vi "Database Recordset Upadate.vi"(8 "error in (no error)":errorcluster caption="错误输入（无错误）", 9 "Values":variant, 10 "Fields":variant, 11 "Database Recordset 输入":refnum<class "Database Recordset.lvclass"> caption="DNL_LabVIEW Object in") -> (0 "error out":errorcluster caption="错误输出", 3 "Database Recordset 输出":refnum<class "Database Recordset.lvclass"> caption="DNL_LabVIEW Object out")   [LabVIEW 2011, in "Database Recordset.lvclass"]
uses:
  Database Recordset.lvclass
  Database Recordset.lvclass/Database Recordset.ctl
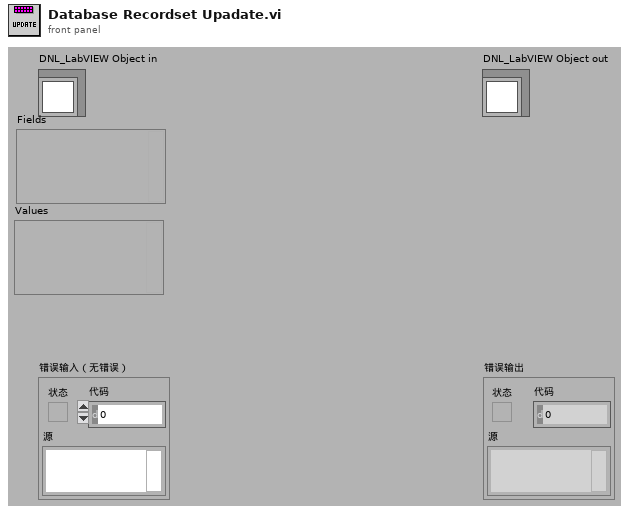
[diagram p1: front panel]
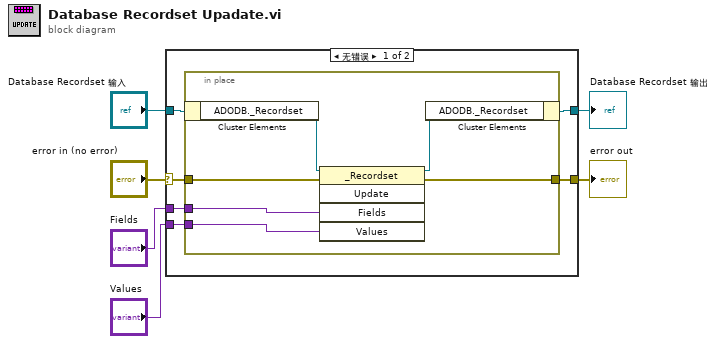
[diagram p0: block diagram]
diagram:
  n1 = case shown="无错误" "error in (no error)" {
    selector: "error in (no error)" -> [w8 w20]
    tunnel: [w7 w20] -> w5
    tunnel: [w9 w19] -> w3
    tunnel: "Database Recordset 输入" -> [w12 w19]
    tunnel: "Fields" -> [w11 _]
    tunnel: "Values" -> [w10 _]
    frame No Error {
      n2 = in-place {
        in-place-border: w11 -> [w16]
        in-place-border: w10 -> [w15]
        in-place-border: w8 -> [w14]
        in-place-border: [w13] -> w7
        n3 = in-place-cluster #1(w12) -> ("ADODB._Recordset"=w18:refnum<k7>)
        n4 = invoke class="_Recordset" method="Update"(reference=w18, error in=w14, "Fields"=w16, "Values"=w15) -> (reference out=w17:refnum<k7>, error out=w13:errorcluster)  [unwired: 1 in, 3 out]
        n5 = in-place-cluster #1("ADODB._Recordset"=w17) -> (w9:refnum<class "Database Recordset.lvclass">)
      }
    }
    frame Error {
    }
  }
  "error out" <- w5
  "Database Recordset 输出" <- w3
